vi "PicIcon.vi"(8 "error in (no error)":errorcluster caption="错误输入（无错误）", 9 "Origin":T1, 10 "Size":T2, 11 "FilePath":path caption="JPEG文件路径") -> (0 "error out":errorcluster caption="错误输出", 2 "IconClass":T4 caption="用户图层")   [LabVIEW 2015]
uses:
  <vilib>/LabVIEW Icon API/API_User Layer Data.ctl
  <vilib>/Utility/miscctls.llb/LVPoint32TypeDef.ctl
  <vilib>/picture/picture.llb/imagedata.ctl
  <vilib>/Utility/miscctls.llb/LVBoundsTypeDef.ctl
  <vilib>/LabVIEW Icon API/LabVIEW Icon API.lvlib
panel:
  out "image data":T3 caption="图像数据"
  out "new picture":picture caption="新图片"
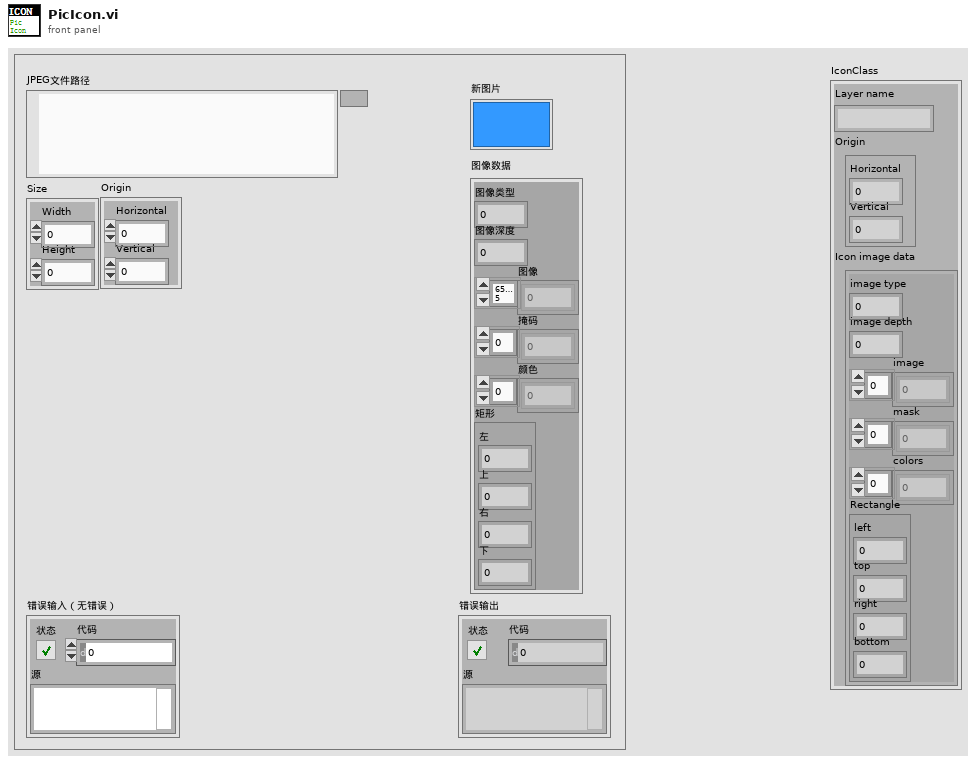
[diagram p1: front panel]
types:
  T1 = typedef "LVPoint32TypeDef.ctl" = cluster{"Horizontal":i32, "Vertical":i32}
  T2 = typedef "LVBoundsTypeDef.ctl" = cluster{"Width":u32, "Height":u32}
  T3 = typedef "imagedata.ctl" = cluster{"image type":i32, "image depth":i32, "image":u8[], "mask":u8[], "colors":u32[], "Rectangle":cluster{"left":i16, "top":i16, "right":i16, "bottom":i16}}
  T4 = typedef "LabVIEW Icon API.lvlib/API_User Layer Data.ctl" = cluster{"Layer name":string, "Origin":T1, "Icon image data":T3}
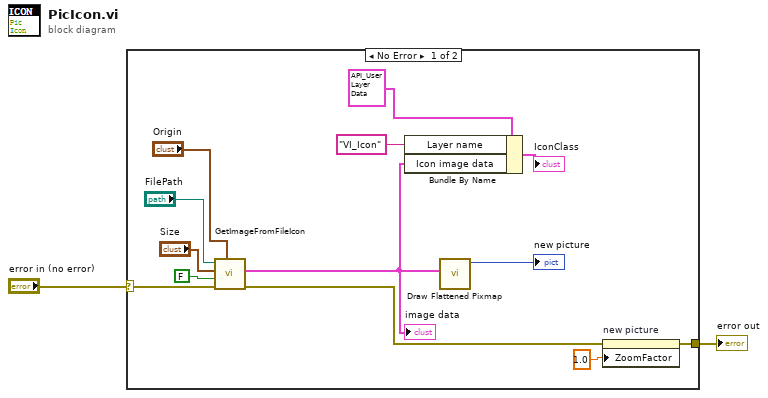
[diagram p0: block diagram]
diagram:
  n1 = case shown="No Error" "error in (no error)" {
    selector: "error in (no error)" -> [w4 w16]
    tunnel: [w5 w16] -> w2
    frame No Error {
      n2 = call "GetImageFromFileIcon.vi"("Origin"="Origin", "error in (no error)"=w4, "AddFrame"=FALSE, "Bounds"="Size", "path to JPEG file"="FilePath") -> ("error out"=w6:errorcluster, "Image Data"=w10:T3)  [unwired: 4 in, 1 out]
      "image data" <- w10
      n3 = Bundle By Name(cluster=T4 {"Layer name"="", "Origin"={"Horizontal"=0, "Vertical"=0}, "Icon image data"={"image type"=0, "image depth"=0, "image"=[], "mask"=[], "colors"=[], "Rectangle"={"left"=0, "top"=0, "right"=0, "bottom"=0}}} ("User layer"), "Layer name"="VI_Icon", "Icon image data"=w10) -> (→"IconClass":T4)
      n4 = call <vilib>:"Draw Flattened Pixmap.vi"("image data"=w10) -> ("new picture"=→"new picture":picture)  [unwired: 8 in]
      n5 = property on="new picture" class="Pict"(error in=w6, "ZoomFactor"=sgl 1.0 ("Zoom Factor")) -> (error out=w5:errorcluster)  [unwired: 1 in, 1 out]
    }
    frame Error {
    }
  }
  "error out" <- w2
